vi "Armed Response.vi"(8 "error in (no error)":errorcluster, 9 "Armed":bool, 10 "Sender":string, 11 "Process Controller in":refnum<class "Process Controller.lvclass">) -> (0 "error out":errorcluster, 3 "Process Controller out":refnum<class "Process Controller.lvclass">)   [LabVIEW 2021]
uses:
  Process Controller.lvclass
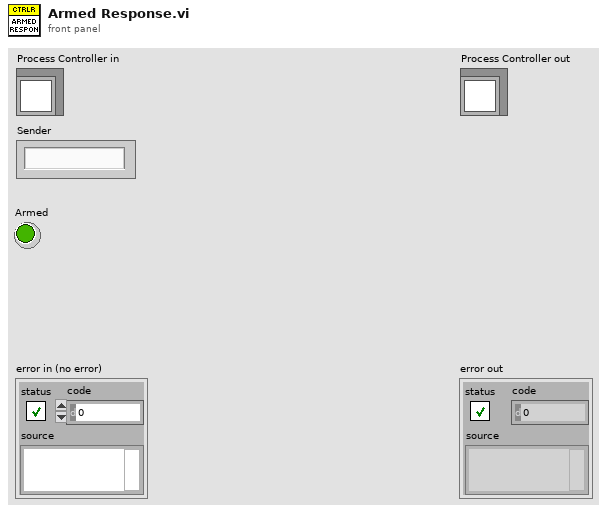
[diagram p1: front panel]
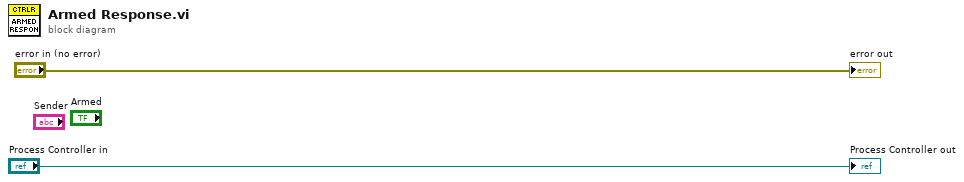
[diagram p0: block diagram]
diagram:
  "error out" <- "error in (no error)"
  "Process Controller out" <- "Process Controller in"
